vi "Agilent 34970 Switch.vi"() -> ()   [LabVIEW 2012]
doc: "This VI shows you how to use the HP34903A GP or the Switch. This example is also valid for the 34901A.\n\nFirst, select the channel(s) you wish to close. Do this by pressing down the button(s) corresponding to the desired channel(s). Then, press the run button on the LabVIEW toolbar.\n\nAny channel whose button is not pressed down will be opened."
uses:
  <instrlib>/Agilent 34970/Agilent 34970.lvlib
panel:
  in  "Module Type":enum16{"34901A or 34903A", "34902A"}(ring)
  in  "Serial Port Configuration":T1={"Timeout Value (10000)"=10000, "Baud Rate (57600)"=enum."57600", "Flow Control (1:XON/XOFF)"=enum."XON / XOFF"}
  in  "Reset (T: Reset)":bool=TRUE
  in  "VISA resource name":refnum<visa-resource-name>
  in  "Channels (F = open)":bool[][](array[boolean])=[[FALSE, FALSE, FALSE, FALSE, FALSE, FALSE, FALSE, FALSE, FALSE, FALSE], [FALSE, FALSE, FALSE, FALSE, FALSE, FALSE, FALSE, FALSE, FALSE, FALSE]]
  in  "Slot Number":u8=1 min=1 max=3 step=1
  # "(c) 2005-2010 National Instruments.  ALL RIGHTS RESERVED."
  # "This Example VI demonstrates using the switching abilities of the HP34970A.  The 34901A and 34903A both have 20 multiplexed channels that can be individually controlled by using the LEDs above.  Setting a LED to off (False) will open the channel.  The  34902A has two 8 channel banks, therefore LED number 9,10,19, and 20 are ignored.\n\nUse the Slot Number control to choose which of the three module slots to access.  Use the Module Type control to specify the what module type is in the slot you have chosen."
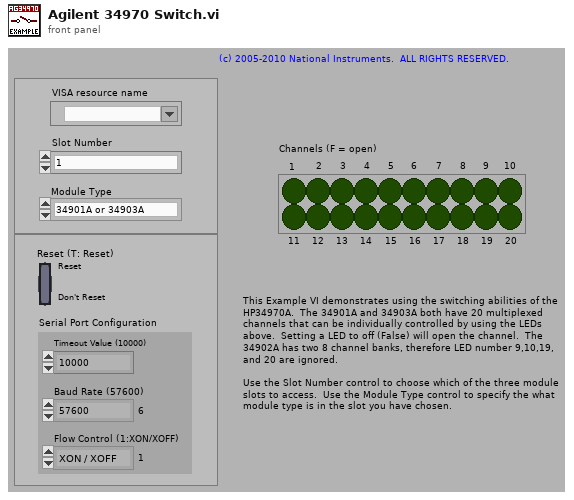
[diagram p1: front panel]
types:
  T1 = cluster{"Timeout Value (10000)":u32, "Baud Rate (57600)":enum16{"1200", "2400", "4800", "9600", "19200", "38400", "57600", "115200"}, "Flow Control (1:XON/XOFF)":enum16{"None", "XON / XOFF", "RTS / CTS", "DTR / DSR"}}
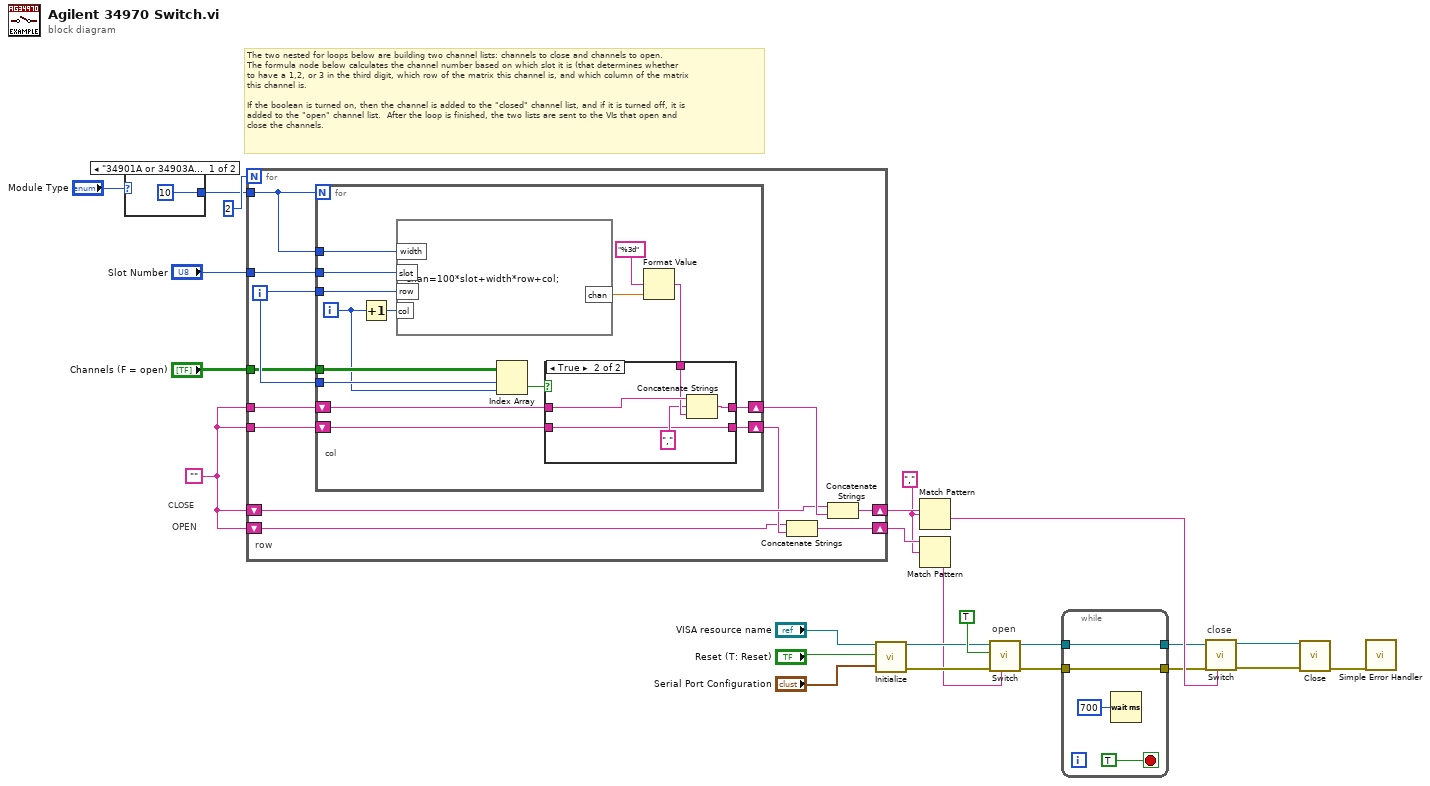
[diagram p0: block diagram]
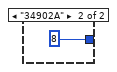
[diagram p2: hidden frame]
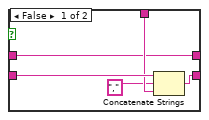
[diagram p3: hidden frame]
diagram:
  w19 = "," ("output string")
  w22 = "" ("Empty String Constant")
  # "The two nested for loops below are building two channel lists: channels to close and channels to open.\nThe formula node below calculates the channel number based on which slot it is (that determines whether\nto have a 1,2, or 3 in the third digit, which row of the matrix this channel is, and which column of the matrix\nthis channel is.\n\nIf the boolean is turned on, then the channel is added to the \"closed\" channel list, and if it is turned off, it is\nadded to the \"open\" channel list.  After the loop is finished, the two lists are sent to the VIs that open and \nclose the channels."
  # "close"
  # "open"
  # "OPEN"
  # "CLOSE"
  n1 = case shown="\"34901A or 34903A\", Default" "Module Type" {
    tunnel: [10 ("y") 8 ("y")] -> w5
    frame "34901A or 34903A", Default {
    }
    frame "34902A" {
    }
  }
  n2 = for {
    N: 2 ("y") -> [_]
    tunnel: "Slot Number" -> [w28]
    shift-right: [w32] -> w21
    shift-left: w22 -> [w33]
    shift-right: [w31] -> w20
    shift-left: w22 -> [w29]
    tunnel: "Channels (F = open)" -> [w37]
    tunnel: w22 -> [w36]
    tunnel: w22 -> [w35]
    tunnel: w5 -> [w27]
    i -> [w38]
    # "row"
    n3 = for {
      N: w27 -> [_]
      tunnel: w38 -> [w53]
      tunnel: w38 -> [w43]
      tunnel: w37 -> [w52]
      shift-right: [w49] -> w34
      shift-left: w36 -> [w50]
      shift-right: [w47] -> w30
      shift-left: w35 -> [w48]
      tunnel: w28 -> [w42]
      tunnel: w27 -> [w39]
      i -> [w46]
      # "col"
      n4 = Increment(x=w46) -> (x+1=w44:i32)
      n5 = formula code="chan=100*slot+width*row+col;"("slot"=w42, "row"=w43, "col"=w44, "width"=w39) -> ("chan"=w41:dbl)
      n6 = Index Array(array=w52, index (row)=w53, index (col)=w46) -> (element=w51:bool)
      n7 = Format Value(format string="%3d", value (0)=w41) -> (output string=w40:string)  [unwired: 1 in]
      n8 = case shown="True" w51 {
        tunnel: w40 -> [w56 w61]
        tunnel: w50 -> [w54 w63]
        tunnel: [w54 w62] -> w49
        tunnel: w48 -> [w58 w59]
        tunnel: [w57 w59] -> w47
        frame False {
          n9 = Concatenate Strings(w58, "," ("output string"), w56) -> (w57:string)
        }
        frame True {
          n10 = Concatenate Strings(w63, "," ("output string"), w61) -> (w62:string)
        }
      }
    }
    n11 = Concatenate Strings(w29, w30) -> (w31:string)
    n12 = Concatenate Strings(w33, w34) -> (w32:string)
  }
  n13 = call <instrlib>:"Initialize.vi"("VISA Resource Name"="VISA resource name", "Reset (T: Reset)"="Reset (T: Reset)", "Serial Port Configuration"="Serial Port Configuration") -> ("VISA Resource Name Out"=w15:refnum<visa-resource-name>, "error out"=w14:errorcluster)  [unwired: 11 in]
  n14 = Match Pattern(string=w21, regular expression=w19) -> (after substring=w17:string)  [unwired: 1 in, 3 out]
  n15 = Match Pattern(string=w20, regular expression=w19) -> (after substring=w11:string)  [unwired: 1 in, 3 out]
  n16 = call <instrlib>:"Switch.vi"("Channel List(empty)"=w11, "error in (no error)"=w14, "Open/Close (F:Close)"=TRUE ("Open/Close"), "VISA Resource Name"=w15) -> ("error out"=w2:errorcluster, "VISA Resource Name Out"=w4:refnum<visa-resource-name>)  [unwired: 5 in, 1 out]
  n17 = while {
    tunnel: [w67] -> w3
    tunnel: w4 -> [w67]
    tunnel: [w66] -> w1
    tunnel: w2 -> [w66]
    stop <- TRUE stop-if-true
    n18 = Wait (ms)(milliseconds to wait=u32 700) -> ()  [unwired: 1 out]
  }
  n19 = call <instrlib>:"Switch.vi"("Channel List(empty)"=w17, "error in (no error)"=w1, "VISA Resource Name"=w3) -> ("error out"=w12:errorcluster, "VISA Resource Name Out"=w13:refnum<visa-resource-name>)  [unwired: 6 in, 1 out]
  n20 = call <instrlib>:"Close.vi"("VISA Resource Name"=w13, "error in (no error)"=w12) -> ("error out"=w10:errorcluster)  [unwired: 13 in]
  n21 = call <vilib>:"Simple Error Handler.vi"("error in (no error)"=w10) -> ()  [unwired: 4 in, 5 out]
